vi "S2DS Edit General Instrument (SubVI).vi"(8 "error in (no error)":errorcluster, 11 "Original Instrument parameters":T1) -> (0 "error out":errorcluster, 3 "Instrument parameters out":T1)   [LabVIEW 2025]
uses:
  TYPE DEFS/S2DS_Instrument parameters.ctl
panel:
  in  "Undo?":bool
  in  "Update?":bool
  in  "Updated Instrument parameters":T1
  # "Update Instrument Parameters..."
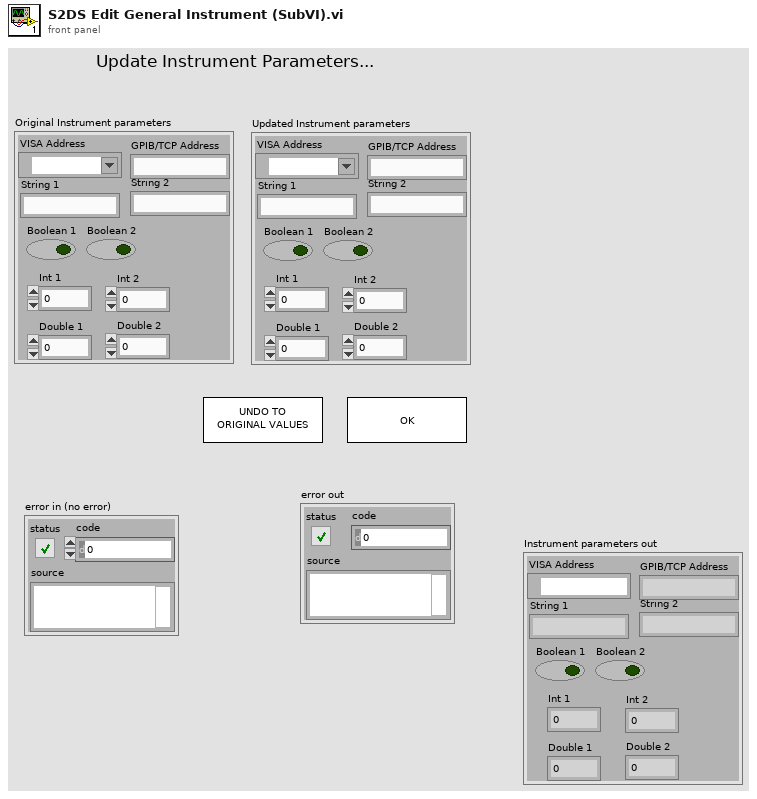
[diagram p1: front panel]
types:
  T1 = typedef "S2DS_Instrument parameters.ctl" = cluster{"VISA Address":refnum<visa-resource-name>, "GPIB/TCP Address":string, "String 1":string, "String 2":string, "Boolean 1":bool, "Boolean 2":bool, "Int 1":i32, "Int 2":i32, "Double 1":dbl, "Double 2":dbl}
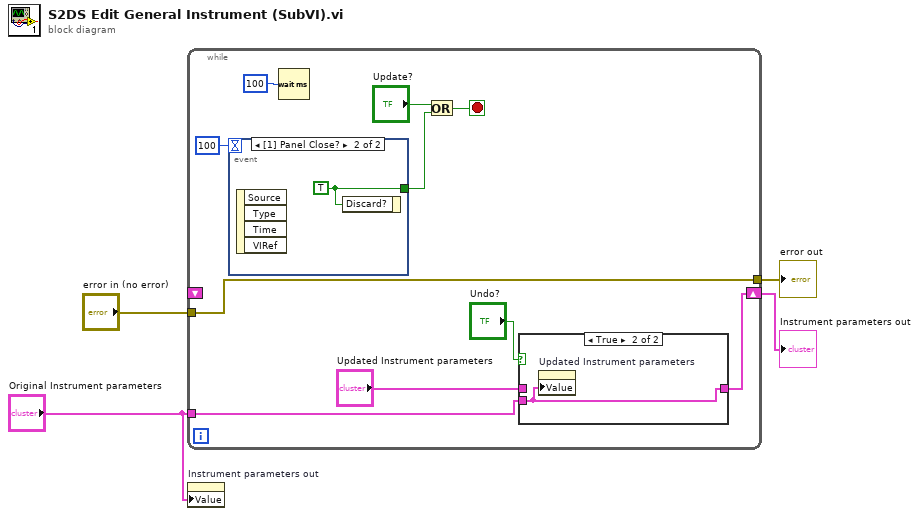
[diagram p0: block diagram]
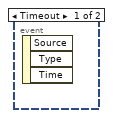
[diagram p3: hidden frame]
diagram:
  n1 = while {
    tunnel: [w14] -> w3
    tunnel: "error in (no error)" -> [w14]
    shift-right: [w7] -> w4
    shift-left: _ -> [_]
    tunnel: "Original Instrument parameters" -> [w8]
    stop <- w10 stop-if-true
    n2 = event shown="[1] Panel Close?" {
      selector: _ -> [_ _]
      dyn-events: _ -> [_ _]
      timeout: 100 -> [_ _]
      tunnel: [_ w17] -> w11
      event Timeout {
        n3 = event-data() -> ()  [unwired: 1 in, 3 out]
      }
      event Panel Close? {
        w17 = TRUE ("Discard?")
        n4 = event-data() -> ()  [unwired: 1 in, 4 out]
        n5 = event-data("Discard?"=w17) -> ()  [unwired: 1 in, 1 out]
      }
    }
    n6 = Wait (ms)(milliseconds to wait=u32 100) -> ()  [unwired: 1 out]
    n7 = Or(x="Update?", y=w11) -> (x .or. y?=w10:bool)
    n8 = case shown="True" "Undo?" {
      tunnel: w8 -> [_ w16]
      tunnel: [w15 w16] -> w7
      tunnel: "Updated Instrument parameters" -> [w15 _]
      frame False {
      }
      frame True {
        n9 = property on="Updated Instrument parameters" class="Clust (strict)"("Value"=w16) -> ()  [unwired: 2 in, 2 out]
      }
    }
  }
  "Instrument parameters out" <- w4
  "error out" <- w3
  n10 = property on="Instrument parameters out" class="Clust (strict)"("Value"="Original Instrument parameters") -> ()  [unwired: 2 in, 2 out]
